vi "PDE_State_Machine_12_12_ver_3.vi"() -> ()   [LabVIEW 2016]
uses:
  PDEState.ctl
  <resource>/objmgr/daqmx.rc
  <vilib>/DAQmx/configure/timing.llb/DAQmx Timing (Sample Clock).vi
  <vilib>/DAQmx/write.llb/DAQmx Write (Digital 1D Wfm NChan NSamp).vi
  <vilib>/DAQmx/create/channels.llb/DAQmx Create Channel (DO-Digital Output).vi
  <vilib>/DAQmx/read.llb/DAQmx Read (Analog 1D Wfm NChan NSamp).vi
  <vilib>/DAQmx/write.llb/DAQmx Write (Digital Wfm 1Chan NSamp).vi
  <vilib>/Waveform/DTblOps.llb/DTbl Boolean Array to Digital.vi
  <vilib>/DAQmx/write.llb/DAQmx Write (Digital Bool 1Line 1Point).vi
  <vilib>/DAQmx/read.llb/DAQmx Read (Analog 1D Wfm NChan 1Samp).vi
  StateIndicator.ctl
  SubVIs/FireSlider.ctl
panel:
  in  "Set_Oxygen_Pressure":bool
  in  "Save Data":bool
  in  "Filename":path=path "test.tdms"
  out "PDE Sensors":T1 {"Downstream Oxygen" scale=0.0..150.0; "Upstream Oxygen" scale=0.0..150.0; "Fuel Pressure" scale=0.0..150.0}
  in  "Predet Freq (Hz)":dbl=20.0 format="%#_13g"
  out "Predet Sensors":T2 {"Fuel Pressure" scale=0.0..150.0; "Oxidizer Pressure" scale=0.0..150.0}
  out "PDE Progress":dbl(slide) scale=0.0..1.0
  out "Predet Progress":dbl(slide) scale=0.0..1.0
  in  "Number of Predet Fires":T3=1 min=0 max=100 step=1 scale=1.0..100.0
  out "Predet Fire Counter":i32
  out "PDE State":T4 items=["Stop VI", "Predet Fire", "Control Button", "Stop", "Connecting", "Firing", "Testing ", "Idle", "Init"]
  in  "Number of Fires":T3=1 min=0 max=100 step=1 scale=1.0..100.0
  out "Fire Counter":i32
  in  "Predet Fire Button":bool
  in  "PDE Fire Button":bool
  in  "Test Button":bool
  in  "Go To Idle":bool
  in  "Abort VI":bool
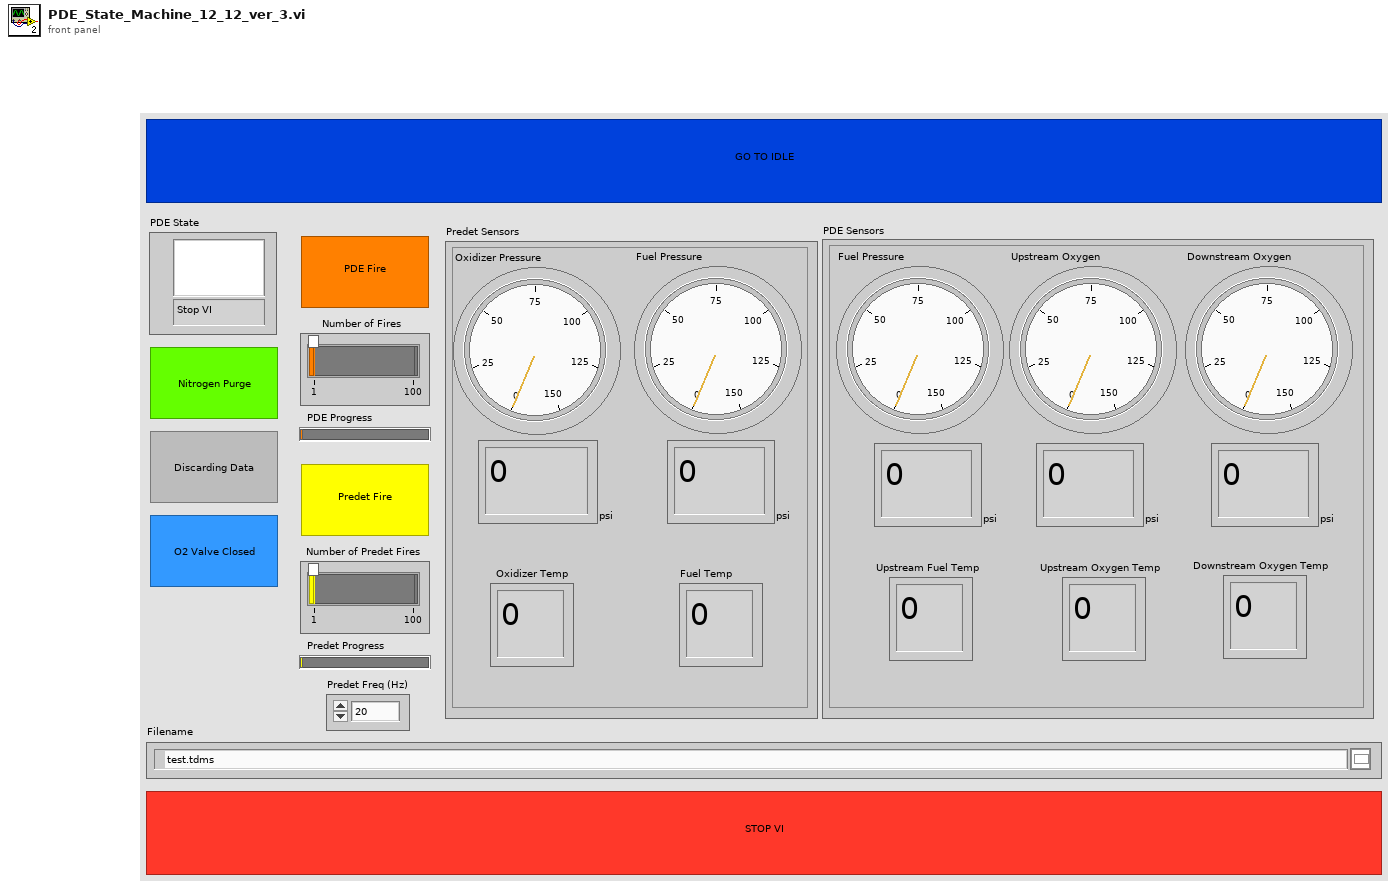
[diagram p1: front panel]
types:
  T1 = cluster{"Fuel Pressure":dbl, "Upstream Oxygen ":dbl, "Downstream Oxygen ":dbl, "Oxidizer Temp":dbl, "Oxidizer Temp 2":dbl, "Oxidizer Temp 3":dbl}
  T2 = cluster{"Oxidizer Pressure":dbl, "Fuel Pressure":dbl, "Oxidizer Temp":dbl, "Fuel Temp":dbl}
  T3 = typedef "FireSlider.ctl" = i32
  T4 = typedef "StateIndicator.ctl" = u16
  T5 = typedef "PDEState.ctl" = enum16{"Stop VI", "Predet Fire", "Control Button", "Stop", "Connecting", "Firing ", "Testing ", "Idle", "Init"}
  T6 = typedef "Rendezvous RefNum" = refnum<k1>
  T7 = cluster{"Scalar":dbl, "Scalar":dbl, "Scalar":dbl, "Scalar":dbl, "Scalar":dbl, "Scalar":dbl}
  T8 = cluster{"Scalar":dbl, "Scalar":dbl, "Scalar":dbl, "Scalar":dbl}
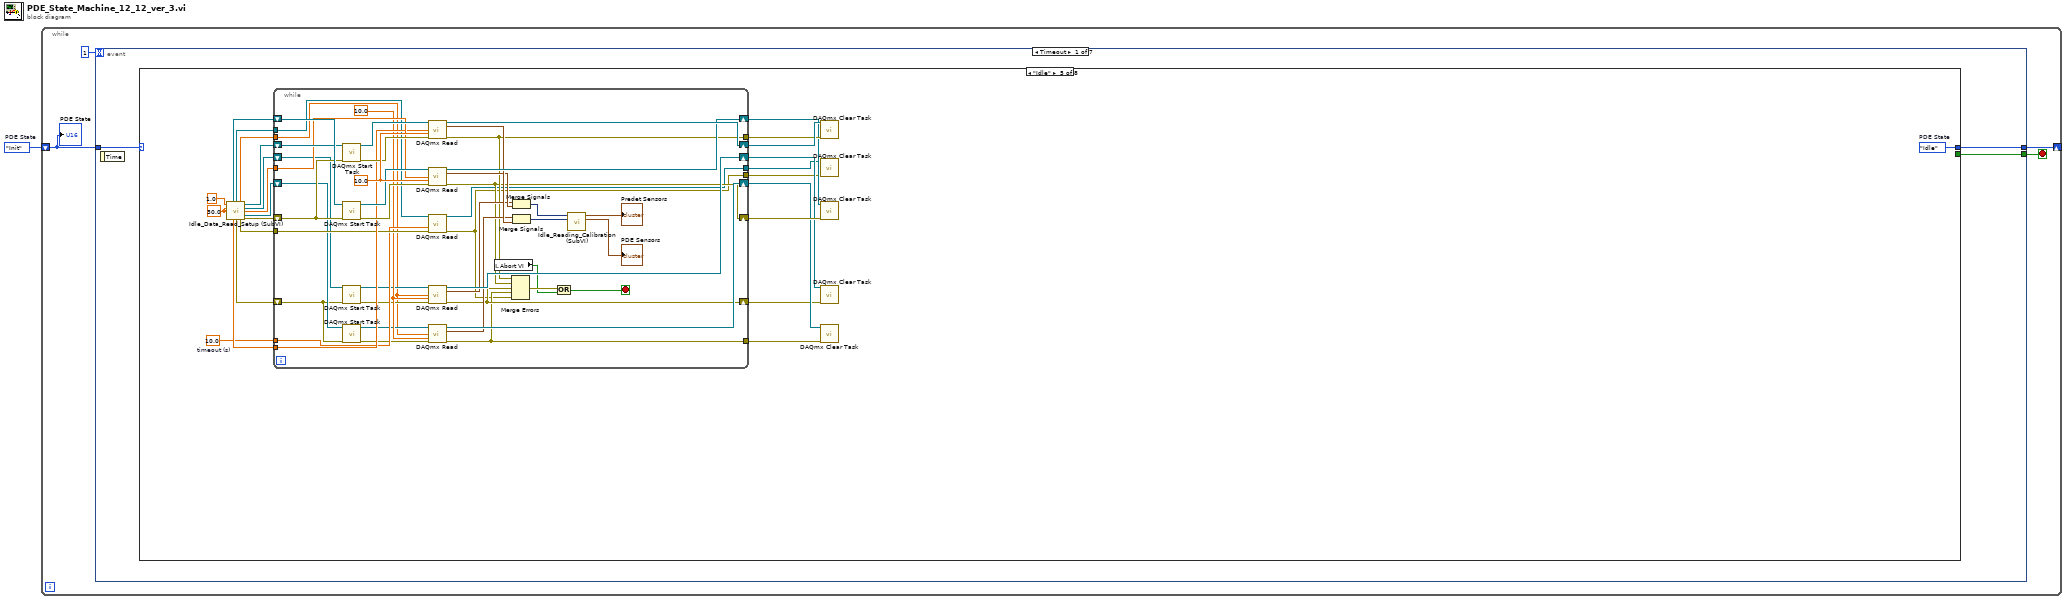
[diagram p0: block diagram]
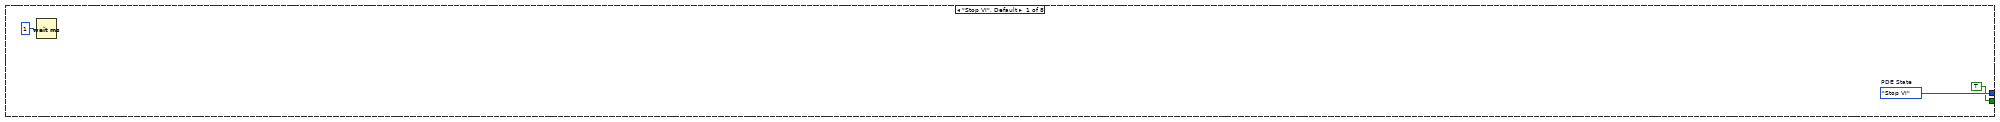
[diagram p2: hidden frame]
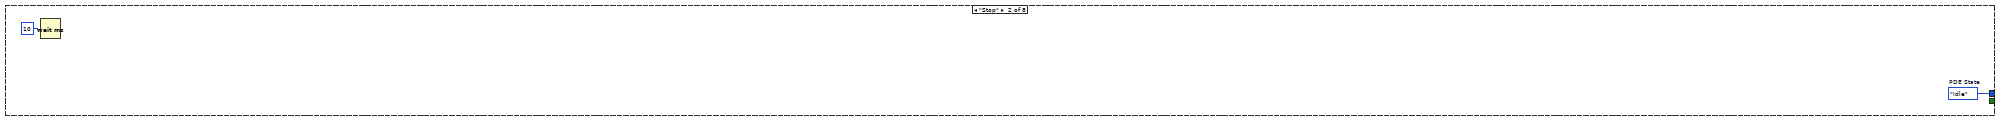
[diagram p3: hidden frame]
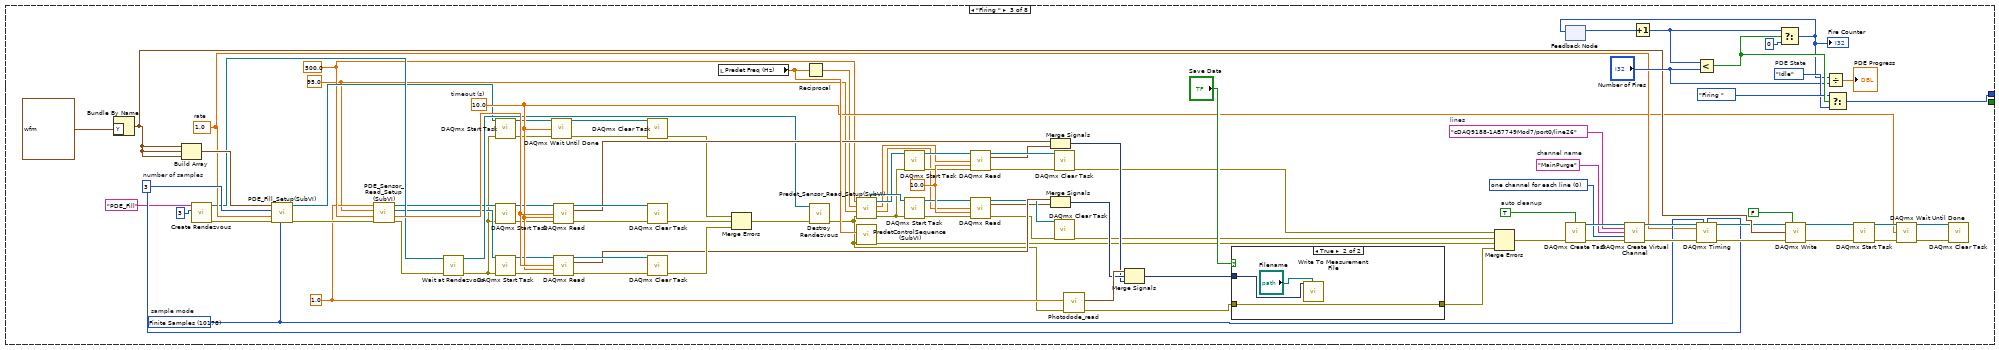
[diagram p4: hidden frame]
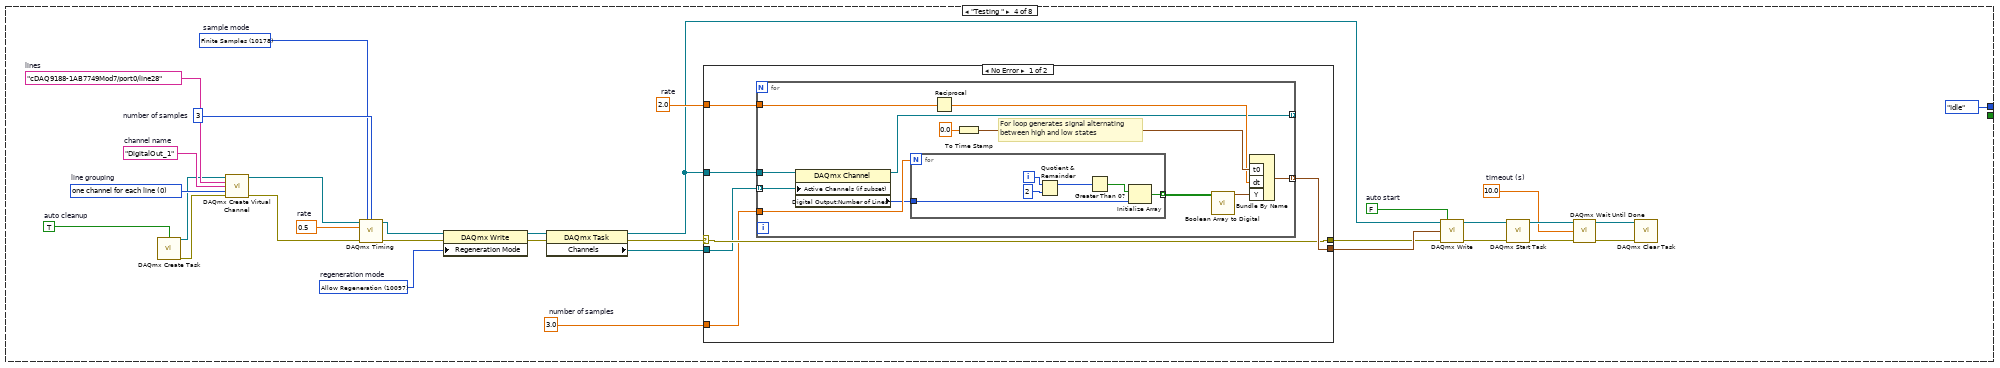
[diagram p6: hidden frame]
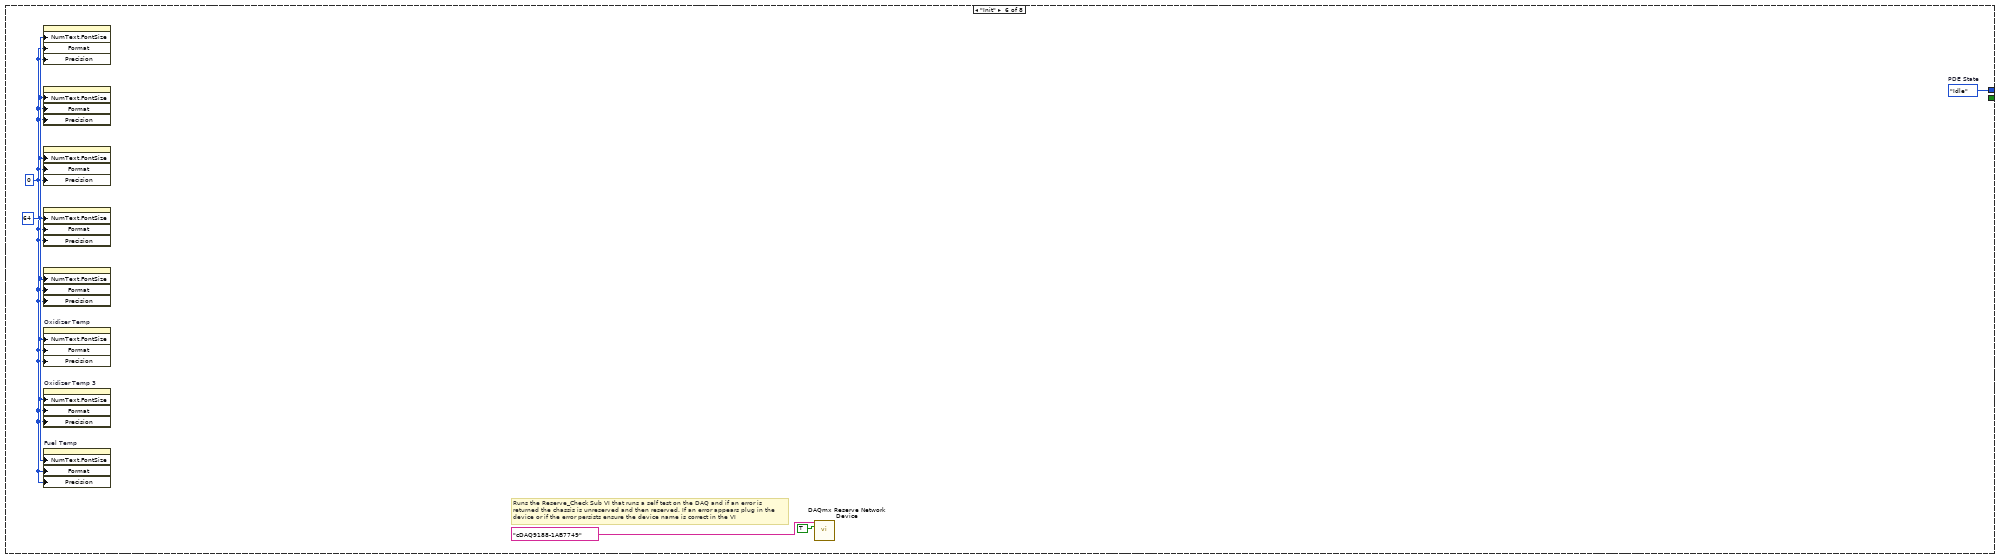
[diagram p8: hidden frame]
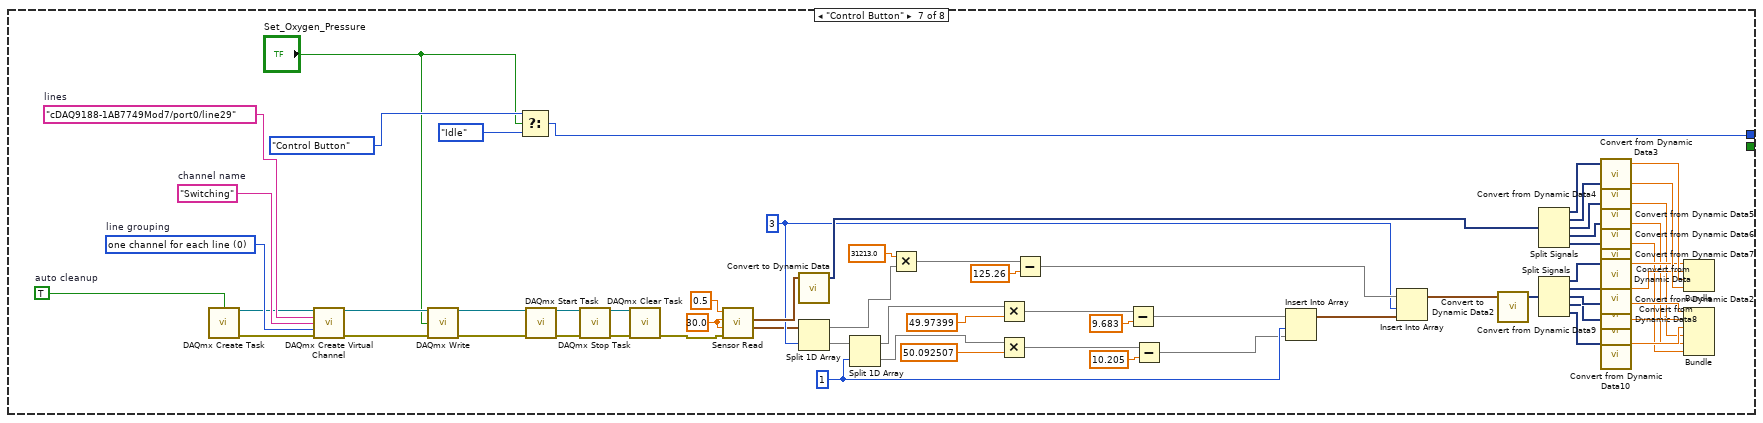
[diagram p9: hidden frame]
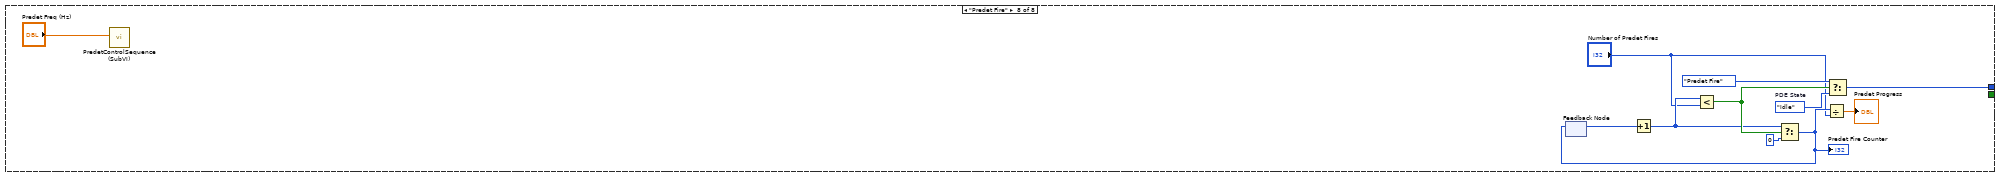
[diagram p10: hidden frame]
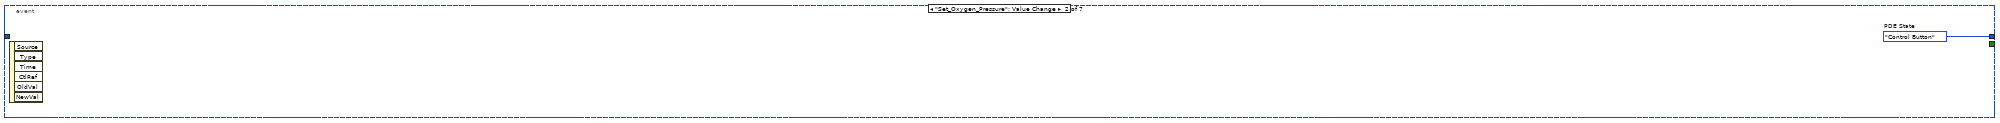
[diagram p11: hidden frame]
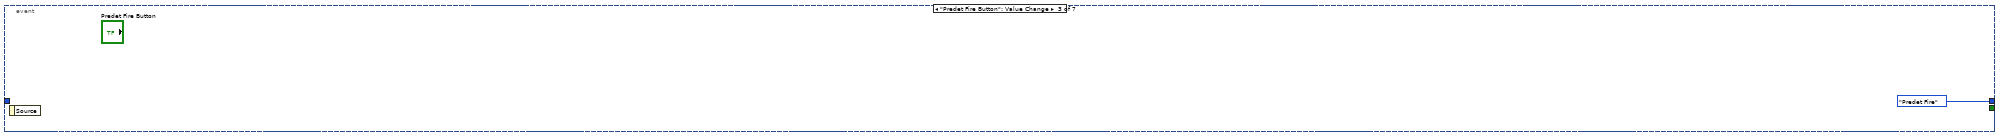
[diagram p12: hidden frame]
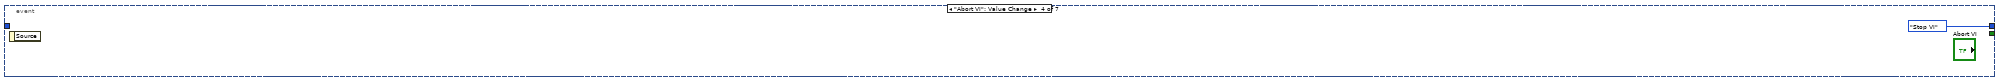
[diagram p13: hidden frame]
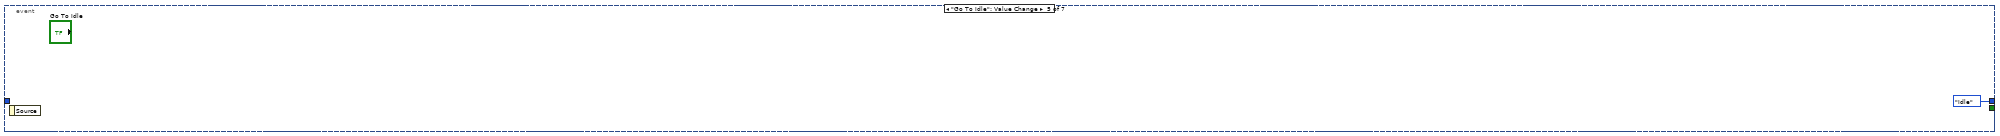
[diagram p14: hidden frame]
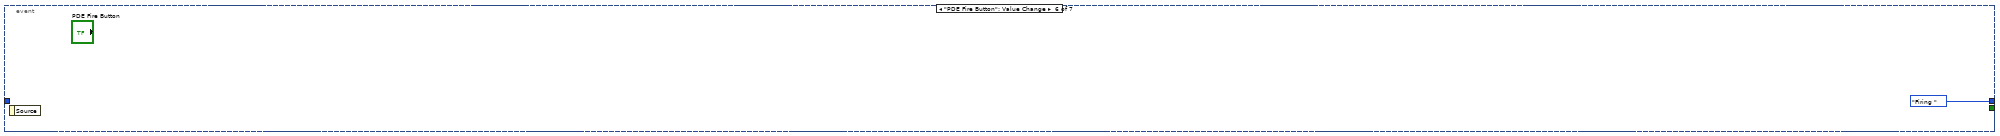
[diagram p15: hidden frame]
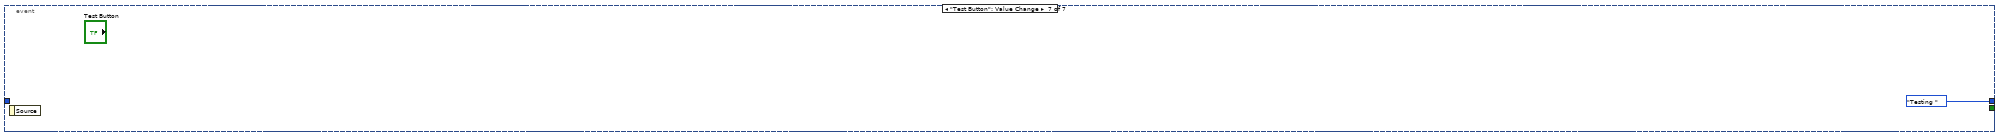
[diagram p16: hidden frame]
diagram:
  w1 = PDEState."Init"  # PDE State
  n1 = while {
    shift-right: [w4] -> _
    shift-left: w1 -> [w2]
    stop <- w3 stop-if-true
    n2 = event shown="[0] Timeout" {
      selector: _ -> [_ _ _ _ _ _ _]
      dyn-events: _ -> [_ _ _ _ _ _ _]
      timeout: 1 -> [_ _ _ _ _ _ _]
      tunnel: w2 -> [w8 _ _ _ _ _ _]
      tunnel: [w7 w321 PDEState."Predet Fire" ("PDE State") PDEState."Stop VI" ("PDE State") PDEState."Idle" ("PDE State") PDEState."Firing " ("PDE State") PDEState."Testing " ("PDE State")] -> w4
      tunnel: [w6 _ _ _ _ _ _] -> w3
      event Timeout {
        n3 = event-data() -> ()  [unwired: 1 in, 1 out]
        n4 = case shown="\"Idle\"" w8 {
          tunnel: [w11 w13 w106 PDEState."Idle" ("PDE State") w196 w244 w308 w314] -> w7
          tunnel: [TRUE _ _ _ _ _ _ _] -> w6
          frame "Stop VI", Default {
            w11 = PDEState."Stop VI"  # PDE State
            n5 = Wait (ms)(milliseconds to wait=u32 1 ("millisecond timer value")) -> ()  [unwired: 1 out]
          }
          frame "Stop" {
            w13 = PDEState."Idle"  # PDE State
            n6 = Wait (ms)(milliseconds to wait=u32 10 ("millisecond timer value")) -> ()  [unwired: 1 out]
          }
          frame "Firing " {
            w41 = 10.0 ("timeout")
            w24 = 1.0 ("Sampling Time")
            w23 = 95.0 ("Temperature Freq")
            w25 = 500.0 ("Pressure Freq")
            w86 = 0 items=["one channel for each line", "one channel for all lines"] ("line grouping")
            w99 = TRUE  # auto cleanup
            w94 = "MainPurge"  # channel name
            w95 = "cDAQ9188-1AB7749Mod7/port0/line26"  # lines
            w79 = 10178 items=["Finite Samples"=10178, "Continuous Samples"=10123, "Hardware Timed Single Point"=12522]  # sample mode
            w80 = 3  # number of samples
            w78 = 1.0  # rate
            w59 = 10.0  # timeout (s)
            w107 = PDEState."Idle"  # PDE State
            n7 = Bundle By Name("Y"=digitaldata {"transitions"=[], "data"=[[0], [1], [0]]}) -> (w85:digitalwaveform)  [unwired: 1 in]
            n8 = Build Array(w85, w85, w85) -> (w100:digitalwaveform[])
            n9 = call <vilib>:"Create Rendezvous.vi"("size (2)"=3, "name (unnamed)"="PDE_Fill") -> ("error out"=w43:errorcluster, "rendezvous"=w56:T6)  [unwired: 3 in, 1 out]
            n10 = call "PDE_Fill_Setup(SubVI).vi"("sample mode"=w79, "Error In"=w43, "rate"=w78, "number of samples"=w80, "Input Boolean Array"=w100) -> ("error out"=w45:errorcluster, "Refnum out"=w52:refnum<k21>)  [unwired: 5 in]
            n11 = call "PDE_Sensor_Read_Setup (SubVI).vi"("Error In"=w45, "Pressure Freq"=w25, "Temperature Freq"=w23, "Sampling Time"=w24) -> ("error out"=w42:errorcluster, "Samples Per Channel"=w62:dbl, "Pressure Task"=w54:refnum<k21>, "Temperature Task"=w53:refnum<k21>)  [unwired: 4 in]
            n12 = call <vilib>:"Wait at Rendezvous.vi"("error in (no error)"=w42, "rendezvous"=w56) -> ("error out"=w44:errorcluster, "rendezvous out"=w55:T6)  [unwired: 3 in, 1 out]
            n13 = call <vilib>:"DAQmx Start Task.vi"("task/channels in"=w52, "error in"=w44) -> ("task out"=w47:refnum<k21>, "error out"=w46:errorcluster)  [unwired: 12 in]
            n14 = call <vilib>:"DAQmx Start Task.vi"("task/channels in"=w53, "error in"=w44) -> ("task out"=w49:refnum<k21>, "error out"=w48:errorcluster)  [unwired: 12 out]
            n15 = call <vilib>:"DAQmx Start Task.vi"("task/channels in"=w54, "error in"=w44) -> ("task out"=w51:refnum<k21>, "error out"=w50:errorcluster)  [unwired: 12 out]
            n16 = call <vilib>:"DAQmx Wait Until Done.vi"("task/channels in"=w47, "timeout (sec)"=w59, "error in"=w46) -> ("task out"=w98:refnum<k21>, "error out"=w102:errorcluster)  [unwired: 11 in]
            n17 = call-poly <vilib>:"DAQmx Read.vi"("task/channels in"=w49, "number of samples per channel"=w62, "timeout"=w59, "error in"=w48) -> ("task out"=w68:refnum<k21>, "data"=w61:waveform(dbl)[], "error out"=w67:errorcluster)  [unwired: 9 out]
            n18 = call-poly <vilib>:"DAQmx Read.vi"("task/channels in"=w51, "number of samples per channel"=w62, "timeout"=w59, "error in"=w50) -> ("task out"=w66:refnum<k21>, "data"=w60:waveform(dbl)[], "error out"=w65:errorcluster)  [unwired: 9 out]
            n19 = call <vilib>:"DAQmx Clear Task.vi"("task in"=w98, "error in"=w102) -> ("error out"=w18:errorcluster)  [unwired: 13 in]
            n20 = call <vilib>:"DAQmx Clear Task.vi"("task in"=w68, "error in"=w67) -> ("error out"=w63:errorcluster)  [unwired: 13 out]
            n21 = call <vilib>:"DAQmx Clear Task.vi"("task in"=w66, "error in"=w65) -> ("error out"=w64:errorcluster)  [unwired: 13 out]
            n22 = local read "Predet Freq (Hz)"() -> (w74:dbl)
            n23 = Merge Errors(w18, w63, w64) -> (w17:errorcluster)
            n24 = Reciprocal(x=w74) -> (1/x=w22:dbl)
            n25 = call <vilib>:"Destroy Rendezvous.vi"("error in (no error)"=w17, "rendezvous"=w55) -> ("error out"=w19:errorcluster)  [unwired: 4 in, 1 out]
            n26 = call "Predet_Sensor_Read_Setup(SubVI).vi"("Error In"=w19, "Temperature Freq"=w23, "Sampling Time"=w22, "Pressure Freq"=w25) -> ("error out"=w28:errorcluster, "Pressure Samples"=w27:dbl, "Temperature Samples"=w26:dbl, "Temperature Task"=w39:refnum<k21>, "Pressure Task"=w40:refnum<k21>)  [unwired: 3 in]
            n27 = call "PredetControlSequence (SubVI).vi"("Predet Freq (Hz)"=w74, "Error In"=w19) -> ("Error Out"=w16:errorcluster)  [unwired: 8 in]
            n28 = call <vilib>:"DAQmx Start Task.vi"("task/channels in"=w39, "error in"=w28) -> ("task out"=w35:refnum<k21>, "error out"=w36:errorcluster)  [unwired: 12 out]
            n29 = call <vilib>:"DAQmx Start Task.vi"("task/channels in"=w40, "error in"=w28) -> ("task out"=w31:refnum<k21>, "error out"=w32:errorcluster)  [unwired: 12 out]
            n30 = call-poly <vilib>:"DAQmx Read.vi"("task/channels in"=w35, "number of samples per channel"=w26, "timeout"=w41, "error in"=w36) -> ("task out"=w38:refnum<k21>, "data"=w20:waveform(dbl)[], "error out"=w37:errorcluster)  [unwired: 9 out]
            n31 = call-poly <vilib>:"DAQmx Read.vi"("task/channels in"=w31, "number of samples per channel"=w27, "timeout"=w41, "error in"=w32) -> ("task out"=w34:refnum<k21>, "data"=w21:waveform(dbl)[], "error out"=w33:errorcluster)  [unwired: 9 out]
            n32 = Merge Signals(w61, w20) -> (w71:dynamicdata)
            n33 = Merge Signals(w60, w21) -> (w72:dynamicdata)
            n34 = call <vilib>:"DAQmx Clear Task.vi"("task in"=w38, "error in"=w37) -> ("error out"=w29:errorcluster)  [unwired: 13 out]
            n35 = call <vilib>:"DAQmx Clear Task.vi"("task in"=w34, "error in"=w33) -> ("error out"=w30:errorcluster)  [unwired: 13 out]
            n36 = call "Photodode_read.vi"("Error In"=w19, "Sampling Time"=w24) -> ("error out"=w69:errorcluster, "data"=w73:waveform(dbl)[])  [unwired: 6 in]
            n37 = Merge Signals(w73, w72, w71) -> (w70:dynamicdata)
            n38 = case shown="True" "Save Data" {
              tunnel: w70 -> [_ w114]
              tunnel: w69 -> [w111 w112]
              tunnel: [w111 w112] -> w14
              frame False {
              }
              frame True {
                n39 = call "Write To Measurement File"("Signals"=w114, "Filename"="Filename") -> ()  [unwired: 15 in, 3 out]
              }
            }
            n40 = Merge Errors(w29, w30, w16, w14) -> (w15:errorcluster)
            n41 = feedback #1() -> (w76:i32)  [unwired: 1 in]
            n42 = call <vilib>:"DAQmx Create Task.vi"("auto cleanup"=w99, "error in"=w15) -> ("task out"=w97:refnum<k21>, "error out"=w96:errorcluster)  [unwired: 12 in]
            n43 = call-poly <vilib>:"DAQmx Create Virtual Channel.vi"("task in"=w97, "lines"=w95, "name to assign"=w94, "line grouping"=w86, "error in"=w96) -> ("task out"=w84:refnum<k21>, "error out"=w81:errorcluster)  [unwired: 9 in]
            n44 = Increment(x=w76) -> (x+1=w77:i32)
            n45 = Less?(x=w77, y="Number of Fires") -> (x < y?=w110:bool)
            n46 = call-poly <vilib>:"DAQmx Timing.vi"("task/channels in"=w84, "sample mode"=w79, "samples per channel"=w80, "rate"=w78, "error in"=w81) -> ("task out"=w83:refnum<k21>, "error out"=w82:errorcluster)  [unwired: 9 in]
            n47 = Select(t=w77, s=w110, f=0 ("s? t:f")) -> (s? t:f=w104:i32)
            "Fire Counter" <- w104
            n48 = feedback-in #1(w104) -> ()
            n49 = call-poly <vilib>:"DAQmx Write.vi"("task/channels in"=w83, "auto start"=FALSE, "data"=w85, "error in"=w82) -> ("task out"=w87:refnum<k21>, "error out"=w88:errorcluster)  [unwired: 9 in, 1 out]
            n50 = Divide(x=w104, y="Number of Fires") -> (x/y=→"PDE Progress":dbl)
            n51 = Select(t=PDEState."Firing ", s=w110, f=w107) -> (s? t:f=w106:T5)
            n52 = call <vilib>:"DAQmx Start Task.vi"("task/channels in"=w87, "error in"=w88) -> ("task out"=w90:refnum<k21>, "error out"=w92:errorcluster)  [unwired: 12 in]
            n53 = call <vilib>:"DAQmx Wait Until Done.vi"("task/channels in"=w90, "timeout (sec)"=w59, "error in"=w92) -> ("task out"=w89:refnum<k21>, "error out"=w91:errorcluster)  [unwired: 11 in]
            n54 = call <vilib>:"DAQmx Clear Task.vi"("task in"=w89, "error in"=w91) -> ()  [unwired: 13 in, 1 out]
          }
          frame "Testing " {
            w126 = 10097 items=["Allow Regeneration"=10097, "Do Not Allow Regeneration"=10158]  # regeneration mode
            w128 = 10178 items=["Finite Samples"=10178, "Continuous Samples"=10123, "Hardware Timed Single Point"=12522]  # sample mode
            w129 = 3  # number of samples
            w130 = 0.5  # rate
            w135 = 0 items=["one channel for each line", "one channel for all lines"]  # line grouping
            w134 = "DigitalOut_1"  # channel name
            w136 = "cDAQ9188-1AB7749Mod7/port0/line28"  # lines
            w137 = TRUE  # auto cleanup
            w138 = 10.0  # timeout (s)
            w122 = 2.0  # rate
            w123 = 3.0  # number of samples
            w145 = FALSE  # auto start
            n55 = call <vilib>:"DAQmx Create Task.vi"("auto cleanup"=w137) -> ("task out"=w116:refnum<k21>, "error out"=w115:errorcluster)  [unwired: 13 in]
            n56 = call-poly <vilib>:"DAQmx Create Virtual Channel.vi"("task in"=w116, "lines"=w136, "name to assign"=w134, "line grouping"=w135, "error in"=w115) -> ("task out"=w131:refnum<k21>, "error out"=w133:errorcluster)  [unwired: 9 in]
            n57 = call-poly <vilib>:"DAQmx Timing.vi"("task/channels in"=w131, "sample mode"=w128, "samples per channel"=w129, "rate"=w130, "error in"=w133) -> ("task out"=w127:refnum<k21>, "error out"=w132:errorcluster)  [unwired: 9 in]
            n58 = property class="DAQmx Write"(reference=w127, error in=w132, "Regeneration Mode"=w126) -> (reference out=w119:refnum<k21>, error out=w118:errorcluster)
            n59 = property class="DAQmx Task"(reference=w119, error in=w118) -> (reference out=w117:refnum<k21>, error out=w124:errorcluster, "Channels"=w125:refnum<k21>[])
            n60 = case shown="No Error" w124 {
              selector: w124 -> [w150 w171]
              tunnel: w122 -> [w152 _]
              tunnel: [w151 _] -> w121
              tunnel: [w150 w171] -> w120
              tunnel: w123 -> [w149 _]
              tunnel: w125 -> [w148 _]
              tunnel: w117 -> [w147 _]
              frame No Error {
                n61 = for {
                  tunnel: w152 -> [w164]
                  tunnel: [w159] -> w151 mode=indexing
                  tunnel: w149 -> [w158]
                  tunnel: w148 -> [w156] mode=indexing
                  tunnel: w147 -> [w154]
                  tunnel: [w153] -> _ mode=indexing
                  # "For loop generates signal alternating\nbetween high and low states"
                  n62 = property class="DAQmx Channel"(reference=w154, "Active Channels (if subset)"=w156) -> (reference out=w153:refnum<k21>, "Digital Output:Number of Lines"=w155:u32)  [unwired: 1 in, 1 out]
                  n63 = for {
                    N: w158 -> [_]
                    tunnel: [w165] -> w157 mode=indexing
                    tunnel: w155 -> [w166]
                    i -> [w170]
                    n64 = Quotient & Remainder(x=w170, y=2) -> (x-y*floor(x/y)=w168:i32)  [unwired: 1 out]
                    n65 = Greater Than 0?(x=w168) -> (x > 0?=w167:bool)
                    n66 = Initialize Array(w167, w166) -> (w165:bool[])
                  }
                  n67 = Reciprocal(x=w164) -> (1/x=w160:dbl)
                  n68 = To Time Stamp(1:0.0) -> (0:w162:timestamp)
                  n69 = call-poly <vilib>:"Boolean Array to Digital.vi"("boolean array"=w157) -> ("digital data"=w161:digitaldata)  [unwired: 3 in, 7 out]
                  n70 = Bundle By Name("t0"=w162, "dt"=w160, "Y"=w161) -> (w159:digitalwaveform)  [unwired: 1 out]
                }
              }
              frame Error {
              }
            }
            n71 = call-poly <vilib>:"DAQmx Write.vi"("task/channels in"=w117, "auto start"=w145, "data"=w121, "error in"=w120) -> ("task out"=w141:refnum<k21>, "error out"=w140:errorcluster)  [unwired: 9 in, 1 out]
            n72 = call <vilib>:"DAQmx Start Task.vi"("task/channels in"=w141, "error in"=w140) -> ("task out"=w144:refnum<k21>, "error out"=w143:errorcluster)  [unwired: 12 in]
            n73 = call <vilib>:"DAQmx Wait Until Done.vi"("task/channels in"=w144, "timeout (sec)"=w138, "error in"=w143) -> ("task out"=w139:refnum<k21>, "error out"=w142:errorcluster)  [unwired: 11 in]
            n74 = call <vilib>:"DAQmx Clear Task.vi"("task in"=w139, "error in"=w142) -> ()  [unwired: 13 in, 1 out]
          }
          frame "Idle" {
            w184 = 10.0  # timeout (s)
            w174 = 30.0 ("Pressure Freq")
            w196 = PDEState."Idle"  # PDE State
            n75 = call "Idle_Data_Read_Setup (SubVI).vi"("Sampling Time"=1.0, "Temperature Freq"=w174, "Pressure Freq"=w174) -> ("Pressure Task 2"=w195:refnum<k21>, "task out"=w185:refnum<k21>, "Samples Per Channel"=w177:dbl, "Refnum out"=w194:refnum<k21>, "Pressure Task"=w176:refnum<k21>, "Pressure Samples"=w188:dbl, "Temperature Task"=w183:refnum<k21>, "Temperature Samples"=w187:dbl, 13:"error out"=w178:errorcluster, "error out 2"=w186:errorcluster, 15:"error out"=w189:errorcluster)  [unwired: 2 in]
            n76 = while {
              tunnel: [w205] -> w192
              tunnel: w188 -> [w227]
              tunnel: w187 -> [w226]
              tunnel: w186 -> [w223]
              tunnel: w185 -> [w222]
              tunnel: w184 -> [w221]
              tunnel: [w202] -> w181
              tunnel: w177 -> [w211]
              shift-right: [w231] -> w191
              shift-left: w195 -> [w236]
              shift-right: [w234] -> w193
              shift-left: w194 -> [w235]
              shift-right: [w204] -> w190
              shift-left: w189 -> [w228]
              shift-right: [w218] -> w182
              shift-left: w183 -> [w219]
              shift-right: [w203] -> w179
              shift-left: w178 -> [w212]
              shift-right: [w215] -> w180
              shift-left: w176 -> [w210]
              tunnel: [w199] -> w173
              tunnel: [w198] -> w172
              stop <- w200 stop-if-true
              w220 = 10.0 ("timeout")
              w237 = 10.0 ("timeout")
              n77 = call <vilib>:"DAQmx Start Task.vi"("task/channels in"=w235, "error in"=w228) -> ("task out"=w232:refnum<k21>, "error out"=w233:errorcluster)  [unwired: 12 out]
              n78 = call <vilib>:"DAQmx Start Task.vi"("task/channels in"=w236, "error in"=w228) -> ("task out"=w229:refnum<k21>, "error out"=w230:errorcluster)  [unwired: 12 out]
              n79 = call <vilib>:"DAQmx Start Task.vi"("task/channels in"=w210, "error in"=w212) -> ("task out"=w213:refnum<k21>, "error out"=w214:errorcluster)  [unwired: 12 out]
              n80 = call <vilib>:"DAQmx Start Task.vi"("task/channels in"=w219, "error in"=w212) -> ("task out"=w216:refnum<k21>, "error out"=w217:errorcluster)  [unwired: 12 out]
              n81 = call-poly <vilib>:"DAQmx Read.vi"("task/channels in"=w232, "number of samples per channel"=w226, "timeout"=w237, "error in"=w233) -> ("task out"=w234:refnum<k21>, "data"=w225:waveform(dbl)[], "error out"=w205:errorcluster)  [unwired: 9 out]
              n82 = call-poly <vilib>:"DAQmx Read.vi"("task/channels in"=w229, "number of samples per channel"=w227, "timeout"=w237, "error in"=w230) -> ("task out"=w231:refnum<k21>, "data"=w224:waveform(dbl)[], "error out"=w204:errorcluster)  [unwired: 9 out]
              n83 = call-poly <vilib>:"DAQmx Read.vi"("task/channels in"=w222, "timeout"=w221, "error in"=w223) -> ("task out"=w199:refnum<k21>, "error out"=w198:errorcluster)  [unwired: 10 in, 1 out]
              n84 = call-poly <vilib>:"DAQmx Read.vi"("task/channels in"=w213, "number of samples per channel"=w211, "timeout"=w220, "error in"=w214) -> ("task out"=w215:refnum<k21>, "data"=w208:waveform(dbl)[], "error out"=w203:errorcluster)  [unwired: 9 out]
              n85 = call-poly <vilib>:"DAQmx Read.vi"("task/channels in"=w216, "number of samples per channel"=w211, "timeout"=w220, "error in"=w217) -> ("task out"=w218:refnum<k21>, "data"=w209:waveform(dbl)[], "error out"=w202:errorcluster)  [unwired: 9 out]
              n86 = local read "Abort VI"() -> (w197:bool)
              n87 = Merge Errors(w205, w204, w203, w202, w198) -> (w201:errorcluster)
              n88 = Merge Signals(w208, w224) -> (w207:dynamicdata)
              n89 = Merge Signals(w209, w225) -> (w206:dynamicdata)
              n90 = Or(x=w201, y=w197) -> (x .or. y?=w200:bool)
              n91 = call "Idle_Reading_Calibration (SubVI).vi"("Dynamic Data"=w206, "Dynamic Data 2"=w207) -> ("Cluster"=→"PDE Sensors":T7, "Cluster 2"=→"Predet Sensors":T8)  [unwired: 8 in]
            }
            n92 = call <vilib>:"DAQmx Clear Task.vi"("task in"=w193, "error in"=w192) -> ()  [unwired: 14 out]
            n93 = call <vilib>:"DAQmx Clear Task.vi"("task in"=w173, "error in"=w172) -> ()  [unwired: 13 in, 1 out]
            n94 = call <vilib>:"DAQmx Clear Task.vi"("task in"=w191, "error in"=w190) -> ()  [unwired: 14 out]
            n95 = call <vilib>:"DAQmx Clear Task.vi"("task in"=w180, "error in"=w179) -> ()  [unwired: 14 out]
            n96 = call <vilib>:"DAQmx Clear Task.vi"("task in"=w182, "error in"=w181) -> ()  [unwired: 14 out]
          }
          frame "Init" {
            w240 = u8 0 ("Display Format:Format")
            w241 = u32 64 ("Numeric Text.Font:Size")
            w244 = PDEState."Idle"  # PDE State
            # "Runs the Reserve_Check Sub VI that runs a self test on the DAQ and if an error is returned the chassis is unreserved and then reserved. If an error appears plug in the device or if the error persists ensure the device name is correct in the VI"
            n97 = property class="DigNum (strict)"("NumText.FontSize"=w241, "Format"=w240, "Precision"=w240) -> ()  [unwired: 2 in, 2 out]
            n98 = property class="DigNum (strict)"("NumText.FontSize"=w241, "Format"=w240, "Precision"=w240) -> ()  [unwired: 2 in, 2 out]
            n99 = property class="DigNum (strict)"("NumText.FontSize"=w241, "Format"=w240, "Precision"=w240) -> ()  [unwired: 2 in, 2 out]
            n100 = property class="DigNum (strict)"("NumText.FontSize"=w241, "Format"=w240, "Precision"=w240) -> ()  [unwired: 2 in, 2 out]
            n101 = property class="DigNum (strict)"("NumText.FontSize"=w241, "Format"=w240, "Precision"=w240) -> ()  [unwired: 2 in, 2 out]
            n102 = property on="Oxidizer Temp" class="DigNum (strict)"("NumText.FontSize"=w241, "Format"=w240, "Precision"=w240) -> ()  [unwired: 2 in, 2 out]
            n103 = property on="Oxidizer Temp 3" class="DigNum (strict)"("NumText.FontSize"=w241, "Format"=w240, "Precision"=w240) -> ()  [unwired: 2 in, 2 out]
            n104 = property on="Fuel Temp" class="DigNum (strict)"("NumText.FontSize"=w241, "Format"=w240, "Precision"=w240) -> ()  [unwired: 2 in, 2 out]
            n105 = call <vilib>:"DAQmx Reserve Network Device.vi"("device in"=tag "cDAQ9188-1AB7749", "override reservation?"=TRUE) -> ()  [unwired: 12 in, 2 out]
          }
          frame "Control Button" {
            w260 = 0 items=["one channel for each line", "one channel for all lines"]  # line grouping
            w259 = "Switching"  # channel name
            w261 = "cDAQ9188-1AB7749Mod7/port0/line29"  # lines
            w262 = TRUE  # auto cleanup
            w246 = 30.0 ("Sampling Frequency")
            w271 = 1 ("index")
            w274 = 3 ("index")
            n106 = call <vilib>:"DAQmx Create Task.vi"("auto cleanup"=w262) -> ("task out"=w258:refnum<k21>, "error out"=w257:errorcluster)  [unwired: 13 in]
            n107 = call-poly <vilib>:"DAQmx Create Virtual Channel.vi"("task in"=w258, "lines"=w261, "name to assign"=w259, "line grouping"=w260, "error in"=w257) -> ("task out"=w256:refnum<k21>, "error out"=w255:errorcluster)  [unwired: 9 in]
            n108 = call-poly <vilib>:"DAQmx Write.vi"("task/channels in"=w256, "data"="Set_Oxygen_Pressure", "error in"=w255) -> ("task out"=w253:refnum<k21>, "error out"=w252:errorcluster)  [unwired: 10 in, 1 out]
            n109 = Select(t=PDEState."Control Button" ("PDE State"), s="Set_Oxygen_Pressure", f=PDEState."Idle" ("PDE State")) -> (s? t:f=w308:T5)
            n110 = call <vilib>:"DAQmx Start Task.vi"("task/channels in"=w253, "error in"=w252) -> ("task out"=w248:refnum<k21>, "error out"=w247:errorcluster)  [unwired: 12 in]
            n111 = call <vilib>:"DAQmx Stop Task.vi"("task/channels in"=w248, "error in"=w247) -> ("task out"=w249:refnum<k21>, "error out"=w250:errorcluster)  [unwired: 12 in]
            n112 = call <vilib>:"DAQmx Clear Task.vi"("task in"=w249, "error in"=w250) -> ("error out"=w251:errorcluster)  [unwired: 13 in]
            n113 = call "Sensor Read.vi"("Error In"=w251, "Pressure Freq"=w246, "Temperature Freq"=w246, "Sampling Time"=0.5) -> ("Temperature Data"=w263:waveform(dbl)[], "Photodiode Data"=w296:waveform(dbl)[])  [unwired: 4 in, 2 out]
            n114 = call "Convert to Dynamic Data"("Array of Waveforms"=w296) -> ("Dynamic Data Type"=w297:dynamicdata)  [unwired: 3 in]
            n115 = Split 1D Array(array=w263, index=w274) -> (first subarray=w280:waveform(dbl)[], second subarray=w273:waveform(dbl)[])
            n116 = Split 1D Array(array=w273, index=w271) -> (first subarray=w265:waveform(dbl)[], second subarray=w264:waveform(dbl)[])
            n117 = Multiply(x=31213.0, y=w280) -> (x*y=w306:waveform(dbl)[])
            n118 = Multiply(x=w265, y=49.97399) -> (x*y=w270:waveform(dbl)[])
            n119 = Multiply(x=w264, y=50.092507) -> (x*y=w279:waveform(dbl)[])
            n120 = Subtract(x=w306, y=125.26) -> (x-y=w276:waveform(dbl)[])
            n121 = Subtract(x=w270, y=9.683) -> (x-y=w266:waveform(dbl)[])
            n122 = Subtract(x=w279, y=10.205) -> (x-y=w267:waveform(dbl)[])
            n123 = Insert Into Array(array=w266, index=w271, new element=w267) -> (w272:waveform(dbl)[])
            n124 = Insert Into Array(array=w276, index=w274, new element=w272) -> (w275:waveform(dbl)[])
            n125 = call "Convert to Dynamic Data2"("Array of Waveforms"=w275) -> ("Dynamic Data Type"=w283:dynamicdata)  [unwired: 3 in]
            n126 = Split Signals(w297) -> (w300:dynamicdata, w302:dynamicdata, w295:dynamicdata, w294:dynamicdata, w293:dynamicdata)  [unwired: 5 in]
            n127 = Split Signals(w283) -> (w286:dynamicdata, w285:dynamicdata, w284:dynamicdata, w282:dynamicdata, w281:dynamicdata)  [unwired: 5 in]
            n128 = call "Convert from Dynamic Data3"("Dynamic Data Type"=w300) -> ("Scalar"=w301:dbl)  [unwired: 3 in]
            n129 = call "Convert from Dynamic Data4"("Dynamic Data Type"=w302) -> ("Scalar"=w303:dbl)  [unwired: 3 in]
            n130 = call "Convert from Dynamic Data5"("Dynamic Data Type"=w295) -> ("Scalar"=w289:dbl)  [unwired: 3 in]
            n131 = call "Convert from Dynamic Data6"("Dynamic Data Type"=w294) -> ("Scalar"=w288:dbl)  [unwired: 3 in]
            n132 = call "Convert from Dynamic Data7"("Dynamic Data Type"=w293) -> ("Scalar"=w287:dbl)  [unwired: 3 in]
            n133 = call "Convert from Dynamic Data"("Dynamic Data Type"=w286) -> ("Scalar"=w299:dbl)  [unwired: 3 in]
            n134 = call "Convert from Dynamic Data2"("Dynamic Data Type"=w285) -> ("Scalar"=w298:dbl)  [unwired: 3 in]
            n135 = call "Convert from Dynamic Data8"("Dynamic Data Type"=w284) -> ("Scalar"=w290:dbl)  [unwired: 3 in]
            n136 = call "Convert from Dynamic Data9"("Dynamic Data Type"=w282) -> ("Scalar"=w291:dbl)  [unwired: 3 in]
            n137 = call "Convert from Dynamic Data10"("Dynamic Data Type"=w281) -> ("Scalar"=w292:dbl)  [unwired: 3 in]
            n138 = Bundle("Scalar"=w299, "Scalar"=w298, "Scalar"=w301, "Scalar"=w303) -> ()  [unwired: 1 in, 1 out]
            n139 = Bundle("Scalar"=w290, "Scalar"=w291, "Scalar"=w292, "Scalar"=w289, "Scalar"=w288, "Scalar"=w287) -> ()  [unwired: 1 in, 1 out]
          }
          frame "Predet Fire" {
            w315 = PDEState."Idle"  # PDE State
            n140 = call "PredetControlSequence (SubVI).vi"("Predet Freq (Hz)"="Predet Freq (Hz)") -> ()  [unwired: 9 in, 1 out]
            n141 = feedback #2() -> (w318:i32)  [unwired: 1 in]
            n142 = Increment(x=w318) -> (x+1=w317:i32)
            n143 = Less?(x=w317, y="Number of Predet Fires") -> (x < y?=w320:bool)
            n144 = Select(t=w317, s=w320, f=0 ("s? t:f")) -> (s? t:f=w313:i32)
            "Predet Fire Counter" <- w313
            n145 = feedback-in #2(w313) -> ()
            n146 = Divide(x=w313, y="Number of Predet Fires") -> (x/y=→"Predet Progress":dbl)
            n147 = Select(t=PDEState."Predet Fire", s=w320, f=w315) -> (s? t:f=w314:T5)
          }
        }
      }
      event "Set_Oxygen_Pressure": Value Change {
        w321 = PDEState."Control Button"  # PDE State
        n148 = event-data() -> ()  [unwired: 1 in, 6 out]
      }
      event "Predet Fire Button": Value Change {
        n149 = event-data() -> ()  [unwired: 1 in, 1 out]
      }
      event "Abort VI": Value Change {
        n150 = event-data() -> ()  [unwired: 1 in, 1 out]
      }
      event "Go To Idle": Value Change {
        n151 = event-data() -> ()  [unwired: 1 in, 1 out]
      }
      event "PDE Fire Button": Value Change {
        n152 = event-data() -> ()  [unwired: 1 in, 1 out]
      }
      event "Test Button": Value Change {
        n153 = event-data() -> ()  [unwired: 1 in, 1 out]
      }
    }
    "PDE State" <- w2
  }
